vi "WriterDaemon.vi"(6 "E-Stop DVR":refnum<data-value>, 8 "error in (no error)":errorcluster, 9 "Connected? DVR":refnum<data-value>, 10 "Message Queue":T2, 11 "Writer Parameters":T1={"writer name"="", "reader url"="", "writer buffer size"=-1}) -> (0 "error out":errorcluster)   [LabVIEW 2012, in "NetworkStreamWriter.lvclass"]
doc: "Daemon (running in the background) which consistently checks the internal queue to see if a new value is available. If a new value is available, it is written across the network stream. If the network stream is disconnected, it will attempt to reconnect until the connection is reestablished or the Close method is called.\n\n<b>This VI must be stopped by calling the Close method of the Object which launched it.</b>\n\nJared Kirschner, 2012."
uses:
  NetworkStreamWriter.lvclass
  Shared/TimeStampedMessageQueue.ctl
  Shared/TimeStampedMessage.ctl
  WriterParameters.ctl
  <vilib>/dex/Flush And Wait Empty Condition.ctl
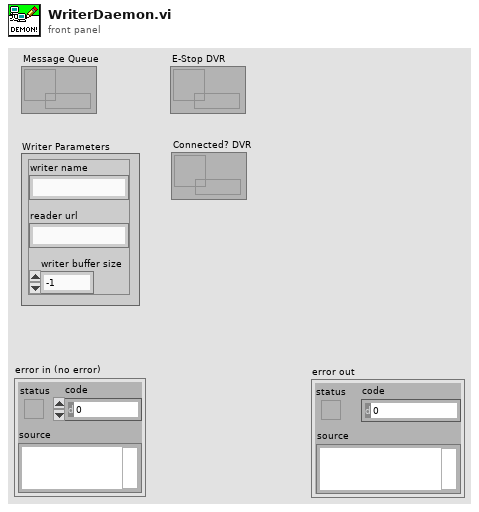
[diagram p1: front panel]
types:
  T1 = typedef "NetworkStreamWriter.lvclass/WriterParameters.ctl" = cluster{"writer name":string, "reader url":string, "writer buffer size":i32}
  T2 = typedef "TimeStampedMessageQueue.ctl" = refnum<queue>
  T3 = typedef "Flush And Wait Empty Condition.ctl" = u8
  T4 = typedef "TimeStampedMessage.ctl" = cluster{"Data":variant, "Time Stamp":timestamp}
  T5 = typedef "ElapsedTimeMessage.ctl" = cluster{"Data":variant, "Elapsed Time (s)":dbl}
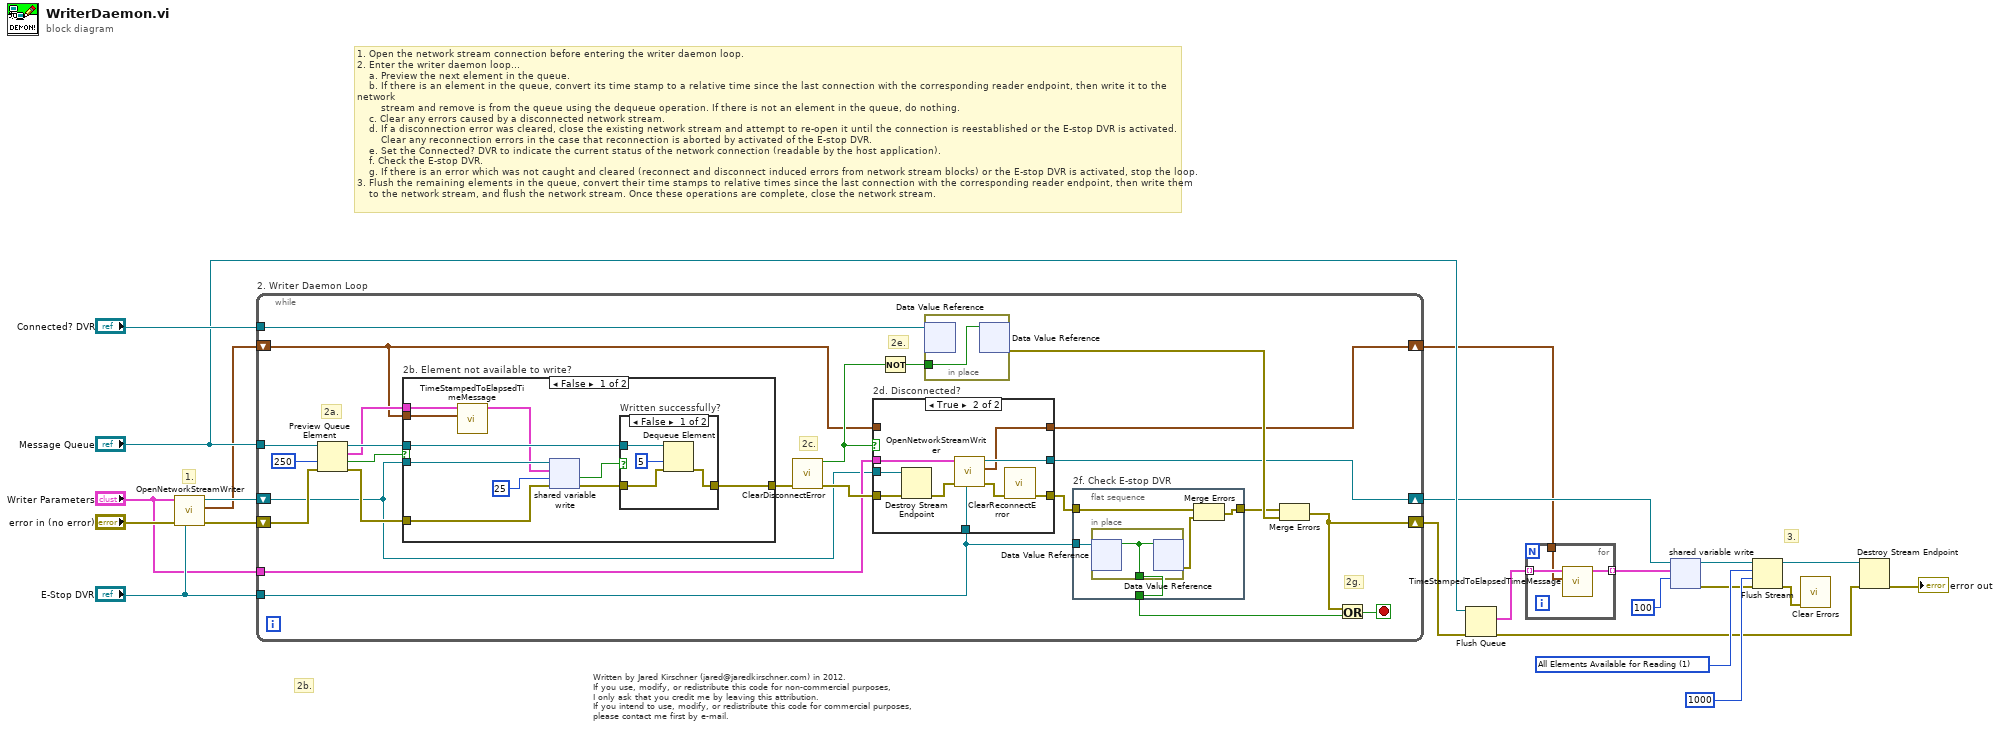
[diagram p0: block diagram]
diagram:
  w22 = T3 1 items=["All Elements Read From Stream", "All Elements Available for Reading"] ("wait condition")
  # "2b."
  # "3."
  # "1."
  # "1. Open the network stream connection before entering the writer daemon loop.\n2. Enter the writer daemon loop...\n    a. Preview the next element in the queue.\n    b. If there is an element in the queue, convert its time stamp to a relative time since the last connection with the corresponding reader endpoint, then write it to the network \n        stream and remove is from the queue using the dequeue operation. If there is not an element in the queue, do nothing.\n    c. Clear any errors caused by a disconnected network stream.\n    d. If a disconnection error was cleared, close the existing network stream and attempt to re-open it until the connection is reestablished or the E-stop DVR is activated.\n        Clear any reconnection errors in the case that reconnection is aborted by activated of the E-stop DVR.\n    e. Set the Connected? DVR to indicate the current status of the network connection (readable by the host application).\n    f. Check the E-stop DVR.\n    g. If there is an error which was not caught and cleared (reconnect and disconnect induced errors from network stream blocks) or the E-stop DVR is activated, stop the loop.\n3. Flush the remaining elements in the queue, convert their time stamps to relative times since the last connection with the corresponding reader endpoint, then write them\n    to the network stream, and flush the network stream. Once these operations are complete, close the network stream."
  # "Written by Jared Kirschner (jared@jaredkirschner.com) in 2012.\nIf you use, modify, or redistribute this code for non-commercial purposes,\nI only ask that you credit me by leaving this attribution.\nIf you intend to use, modify, or redistribute this code for commercial purposes,\nplease contact me first by e-mail."
  n1 = call "OpenNetworkStreamWriter.vi"("E-Stop DVR"="E-Stop DVR", "error in (no error)"="error in (no error)", "Writer Parameters"="Writer Parameters") -> ("error out"=w17:errorcluster, "Time Opened"=w7:timestamp, "Writer Endpoint"=w18:refnum<k21>)  [unwired: 5 in, 1 out]
  n2 = while "2. Writer Daemon Loop" {
    tunnel: "Message Queue" -> [w46]
    shift-right: [w38] -> w11
    shift-left: w17 -> [w42]
    tunnel: "E-Stop DVR" -> [w31]
    tunnel: "Connected? DVR" -> [w37]
    tunnel: "Writer Parameters" -> [w35]
    shift-right: [w34] -> w10
    shift-left: w18 -> [w33]
    shift-right: [w26] -> w4
    shift-left: w7 -> [w24]
    stop <- w40 stop-if-true
    # "2g."
    # "2e."
    # "2c."
    # "2a."
    n3 = Preview Queue Element(queue=w46, timeout in ms (-1)=250, error in (no error)=w42) -> (queue out=w43:T2, element=w25:T4, timed out?=w23:bool, error out=w44:errorcluster)
    n4 = case "2b. Element not available to write?" shown="False" w23 {
      tunnel: w44 -> [w74 w81]
      tunnel: w33 -> [w75 _]
      tunnel: w43 -> [w73 _]
      tunnel: [w71 w81] -> w41
      tunnel: w25 -> [w68 _]
      tunnel: w24 -> [w67 _]
      frame False {
        n5 = call "TimeStampedToElapsedTimeMessage.vi"("Time Opened"=w67, "TimeStampedMessage"=w68) -> ("ElapsedTimeMessage"=w66:T5)  [unwired: 9 in]
        n6 = shared-variable-write(w75, w74, w66, 25 ("timeout ms (-1)")) -> (w72:errorcluster, w69:bool)  [unwired: 1 out]
        n7 = case "Written successfully?" shown="False" w69 {
          tunnel: w73 -> [w79 _]
          tunnel: w72 -> [w78 w80]
          tunnel: [w76 w80] -> w71
          frame False {
            n8 = Dequeue Element(queue=w79, timeout in ms (-1)=5, error in (no error)=w78) -> (error out=w76:errorcluster)  [unwired: 3 out]
          }
          frame True {
          }
        }
      }
      frame True {
      }
    }
    n9 = call "ClearDisconnectError.vi"("error in (no error)"=w41) -> ("error out"=w36:errorcluster, "Disconnect error?"=w28:bool)  [unwired: 9 in]
    n10 = case "2d. Disconnected?" shown="True" w28 {
      tunnel: w36 -> [w55 w61]
      tunnel: [w55 w58] -> w32
      tunnel: w35 -> [_ w64]
      tunnel: [w54 w63] -> w34
      tunnel: w33 -> [w54 w62]
      tunnel: w31 -> [_ w57]
      tunnel: w24 -> [w53 _]
      tunnel: [w53 w56] -> w26
      frame False {
      }
      frame True {
        n11 = Destroy Stream Endpoint(8:w61, 11:w62) -> (0:w60:errorcluster)
        n12 = call "OpenNetworkStreamWriter.vi"("E-Stop DVR"=w57, "error in (no error)"=w60, "Writer Parameters"=w64) -> ("error out"=w59:errorcluster, "Time Opened"=w56:timestamp, "Writer Endpoint"=w63:refnum<k21>)  [unwired: 5 in, 1 out]
        n13 = call "ClearReconnectError.vi"("error in (no error)"=w59) -> ("error out"=w58:errorcluster)  [unwired: 9 in, 1 out]
      }
    }
    n14 = Not(x=w28) -> (.not. x?=w27:bool)
    n15 = in-place {
      in-place-border: w27 -> [w65]
      n16 = in-place-dvr #1(w37) -> ()  [unwired: 2 out]
      n17 = in-place-dvr #1(w65) -> (w39:errorcluster)  [unwired: 1 out]
    }
    n18 = flat-sequence "2f. Check E-stop DVR" {
      tunnel: [w47] -> _
      tunnel: [w51] -> w30
      tunnel: w32 -> [w49]
      tunnel: w31 -> [w48]
      tunnel: [w47] -> w29
      frame #0 {
        n19 = in-place {
          in-place-border: [w52] -> w47
          n20 = in-place-dvr #2(w48) -> (w52:bool)  [unwired: 1 out]
          n21 = in-place-dvr #2(w52) -> (w50:errorcluster)  [unwired: 1 out]
        }
        n22 = Merge Errors(w49, w50) -> (w51:errorcluster)
      }
    }
    n23 = Merge Errors(w30, w39) -> (w38:errorcluster)
    n24 = Or(x=w38, y=w29) -> (x .or. y?=w40:bool)
  }
  n25 = Flush Queue(queue="Message Queue", error in (no error)=w11) -> (remaining elements=w6:T4[], error out=w2:errorcluster)  [unwired: 1 out]
  n26 = for {
    tunnel: w6 -> [w84] mode=indexing
    tunnel: [w83] -> w5 mode=indexing
    tunnel: w4 -> [w82]
    n27 = call "TimeStampedToElapsedTimeMessage.vi"("Time Opened"=w82, "TimeStampedMessage"=w84) -> ("ElapsedTimeMessage"=w83:T5)  [unwired: 9 in]
  }
  n28 = shared-variable-write(w10, w5, 100 ("timeout ms (-1)")) -> (w9:refnum<k21>, w3:errorcluster)  [unwired: 1 in, 1 out]
  n29 = Flush Stream(8:w3, 9:1000 ("timeout in ms (-1)"), 10:w22, 11:w9) -> (0:w1:errorcluster, 3:w20:refnum<k21>)  [unwired: 1 out]
  n30 = call <vilib>:"Clear Errors.vi"("error in (no error)"=w1) -> ()  [unwired: 6 in, 1 out]
  n31 = Destroy Stream Endpoint(8:w2, 11:w20) -> (0:→"error out":errorcluster)
